vi "I_control.vi"(8 "Ki":dbl=10.0 format="%#_13g", 10 "Past measures":dbl[](array[numeric]), 11 "Feedback error":dbl[](array[numeric])) -> (3 "I control":dbl[](array[numeric]))   [LabVIEW 2021]
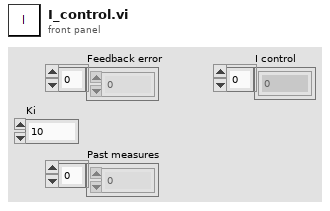
[diagram p1: front panel]
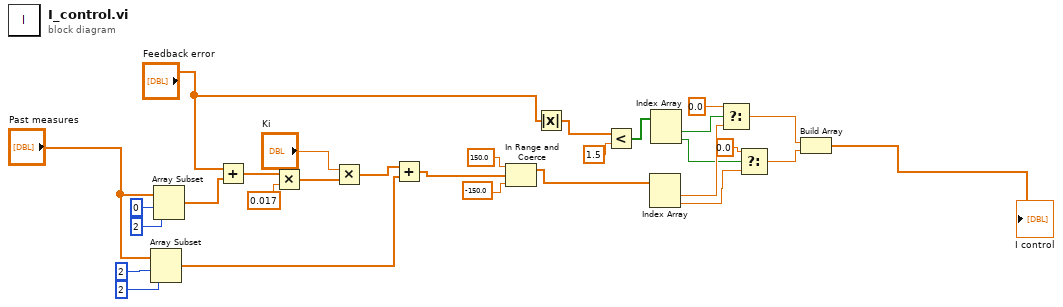
[diagram p0: block diagram]
diagram:
  n1 = Array Subset(array="Past measures", index=2, length=2) -> (w15:dbl[])
  n2 = Array Subset(array="Past measures", index=0, length=2) -> (w17:dbl[])
  n3 = Add(x="Feedback error", y=w17) -> (x+y=w22:dbl[])
  n4 = Multiply(x=w22, y=0.017) -> (x*y=w24:dbl[])
  n5 = Multiply(x="Ki", y=w24) -> (x*y=w26:dbl[])
  n6 = Add(x=w26, y=w15) -> (x+y=w29:dbl[])
  n7 = In Range and Coerce(upper limit=150.0, x=w29, lower limit=-150.0) -> (coerced(x)=w8:dbl[])  [unwired: 1 out]
  n8 = Absolute Value(x="Feedback error") -> (abs(x)=w13:dbl[])
  n9 = Less?(x=w13, y=1.5) -> (x < y?=w11:bool[])
  n10 = Index Array(array=w8) -> (element #1=w7:dbl, element #2=w6:dbl)  [unwired: 2 in]
  n11 = Index Array(array=w11) -> (element #1=w10:bool, element #2=w5:bool)  [unwired: 2 in]
  n12 = Select(t=0.0, s=w10, f=w7) -> (s? t:f=w3:dbl)
  n13 = Select(t=0.0, s=w5, f=w6) -> (s? t:f=w2:dbl)
  n14 = Build Array(w3, w2) -> (→"I control":dbl[])
